vi "Marginal Condition.vi"() -> ()   [LabVIEW 2023]
doc: "This example shows how to compute the marginal condition of a spectrogram with the TFA Marginal Integration VI. The Wigner-Ville distribution (WVD) or Choi-Williams distribution (CWD) of a Gaussian chirp is computed. In theory, the time and frequency marginal conditions of the WVD and CWD are exactly corresponding to the instantaneous power and the FFT-based power spectrum respectively. The example demonstrates such property of the WVD and CWD.\n\n<b>Instructions:</b>\n1) Run this VI.\n2) Compare the <b>Power Spectrum</b> and <b>Instantaneous Power</b> of the simulated signal."
uses:
  <vilib>/Analysis/2dsp.llb/Complex FFT.vi
  <vilib>/addons/Time Frequency Analysis/Spectrogram.llb/TFA Wigner-Ville Distribution (Complex).vi
  <vilib>/addons/Time Frequency Analysis/Spectrogram.llb/TFA Choi-Williams Distribution (Complex).vi
  <vilib>/addons/Time Frequency Analysis/_control.llb/TFA Configure Spectrogram Indicator (Predefined Color Table).vi
  <vilib>/addons/_Advanced Signal Processing/NI_AdvSigProcTFA.lvlib
  <vilib>/Analysis/NI_AALPro.lvlib
panel:
  out "aspt-left-top":bool
  in  "Type":u16(ring) items=["WVD", "CWD"]
  out "Spectrogram":dbl[][](graph)
  out "Signal":cluster{"sampling rate":dbl, dbl, dbl[]}[](graph)
  out "Instantaneous power":cluster{"t0":dbl, "dt":dbl, "power":dbl[]}[](graph)
  out "Power spectrum":cluster{"f0":dbl, "df":dbl, "spectrum":dbl[]}[](graph)
  # "Overview: Shows how to compute the marginal condition of a spectrogram with the TFA Marginal Integration VI. \nRequirements: LabVIEW Full Development System, Advanced Signal Processing Toolkit\nInstructions: \n1. Run this VI.\n2. Compare the Power Spectrum and Instantaneous Power of the simulated signal."
  # "Signal and Spectrogram"
  # "Power Spectrum"
  # "Instantaneous Power"
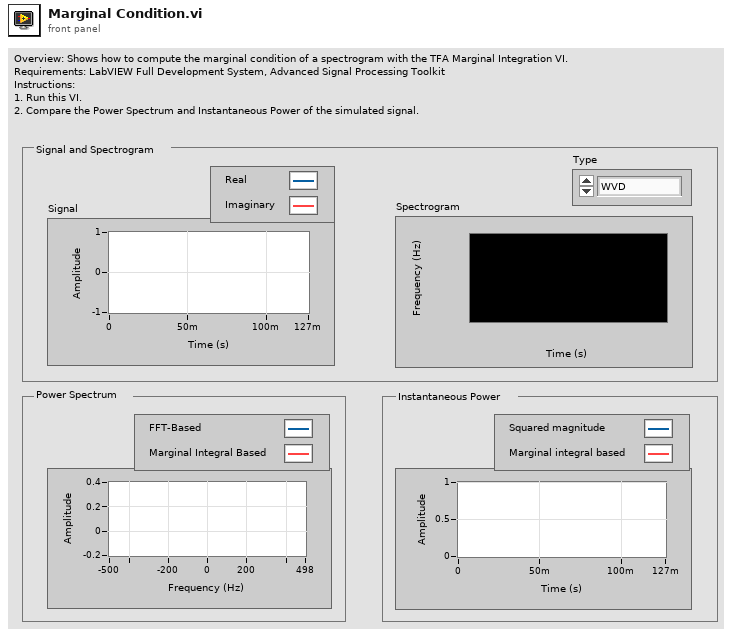
[diagram p1: front panel]
types:
  T1 = cluster{"magnitude":dbl, "phase":dbl, "std dev":dbl, "center":dbl, "frequency":dbl, "chirp rate":dbl}[]
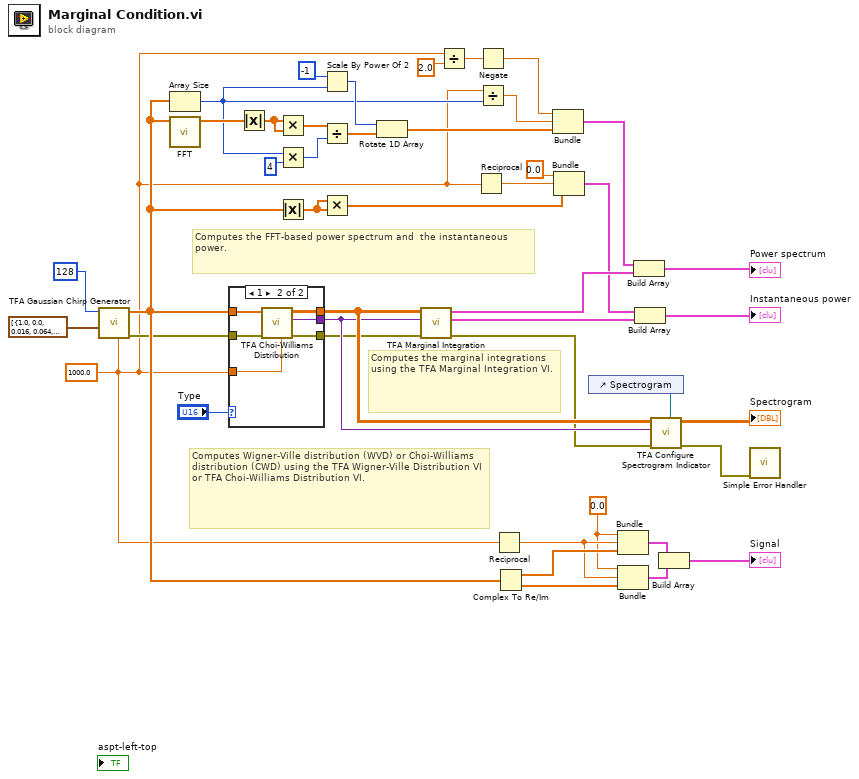
[diagram p0: block diagram]
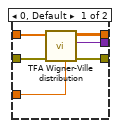
[diagram p2: hidden frame]
diagram:
  w10 = 0.0 ("sampling rate")
  w1 = 1000.0 ("sampling rate")
  # "Computes the marginal integrations using the TFA Marginal Integration VI."
  # "Computes the FFT-based power spectrum and  the instantaneous power."
  # "Computes Wigner-Ville distribution (WVD) or Choi-Williams distribution (CWD) using the TFA Wigner-Ville Distribution VI or TFA Choi-Williams Distribution VI."
  n1 = call <vilib>:"TFA Gaussian Chirp Generator.vi"("sampling rate"=w1, "chirp info"=T1 [{"magnitude"=1.0, "phase"=0.0, "std dev"=0.016, "center"=0.064, "frequency"=100.0, "chirp rate"=5000.0}] ("paras"), "samples"=128) -> ("error out"=w5:errorcluster, "Gaussian chirp"=w7:cdb[])  [unwired: 1 in, 6 out]
  n2 = Array Size(array=w7) -> (size(s)=w26:i32)
  n3 = call-poly <vilib>:"FFT.vi"("X"=w7) -> ("FFT {X}"=w43:cdb[])  [unwired: 2 in, 8 out]
  n4 = case shown="1" "Type" {
    tunnel: w7 -> [w50 w56]
    tunnel: [w49 w55] -> w32
    tunnel: [w48 w54] -> w31
    tunnel: w1 -> [w47 w53]
    tunnel: w5 -> [w46 w52]
    tunnel: [w45 w51] -> w4
    frame 0, Default {
      n5 = call-poly <vilib>:"TFA Wigner-Ville distribution.vi"("sampling rate"=w47, "error in (no error)"=w46, "signal"=w50) -> ("error out"=w45:errorcluster, "scale info"=w48:variant, "spectrogram"=w49:dbl[][])  [unwired: 1 in, 5 out]
    }
    frame 1 {
      n6 = call-poly <vilib>:"TFA Choi-Williams Distribution.vi"("sampling rate"=w53, "error in (no error)"=w52, "signal"=w56) -> ("error out"=w51:errorcluster, "scale info"=w54:variant, "spectrogram"=w55:dbl[][])  [unwired: 2 in, 4 out]
    }
  }
  n7 = Absolute Value(x=w43) -> (abs(x)=w42:dbl[])
  n8 = Multiply(x=w42, y=w42) -> (x*y=w41:dbl[])
  n9 = Multiply(x=w26, y=4) -> (x*y=w38:i32)
  n10 = Absolute Value(x=w7) -> (abs(x)=w44:dbl[])
  n11 = Scale By Power Of 2(n=-1, x=w26) -> (x*2^n=w35:i32)
  n12 = Divide(x=w41, y=w38) -> (x/y=w39:dbl[])
  n13 = Multiply(x=w44, y=w44) -> (x*y=w22:dbl[])
  n14 = Rotate 1D Array(1:w39, 2:w35) -> (0:w27:dbl[])
  n15 = call <vilib>:"TFA Marginal Integration.vi"("error in (no error)"=w4, "scale info"=w31, "spectrogram"=w32) -> ("error out"=w3:errorcluster, "time marginal integral"=w18:cluster{"t0":dbl, "dt":dbl, "power":dbl[]}, "frequency marginal integral"=w40:cluster{"f0":dbl, "df":dbl, "spectrum":dbl[]})  [unwired: 6 out]
  n16 = Divide(x=w1, y=2.0) -> (x/y=w16:dbl)
  n17 = Reciprocal(x=w1) -> (1/x=w21:dbl)
  n18 = Negate(x=w16) -> (-x=w14:dbl)
  n19 = Divide(x=w1, y=w26) -> (x/y=w25:dbl)
  n20 = Reciprocal(x=w1) -> (1/x=w11:dbl)
  n21 = Complex To Re/Im(x + iy=w7) -> (x=w13:dbl[], y=w12:dbl[])
  n22 = Bundle(w14, w25, w27) -> (w23:cluster{dbl, dbl, dbl[]})  [unwired: 1 out]
  n23 = Bundle(0.0, w21, w22) -> (w19:cluster{dbl, dbl, dbl[]})  [unwired: 1 out]
  n24 = control-ref of="Spectrogram"() -> (w29:refnum<vi>)
  n25 = Bundle("sampling rate"=w10, w11, w13) -> (w9:cluster{"sampling rate":dbl, dbl, dbl[]})  [unwired: 1 out]
  n26 = Bundle("sampling rate"=w10, w11, w12) -> (w8:cluster{"sampling rate":dbl, dbl, dbl[]})  [unwired: 1 out]
  n27 = Build Array(w23, w40) -> (→"Power spectrum":cluster{"f0":dbl, "df":dbl, "spectrum":dbl[]}[])
  n28 = Build Array(w19, w18) -> (→"Instantaneous power":cluster{"t0":dbl, "dt":dbl, "power":dbl[]}[])
  n29 = call-poly <vilib>:"TFA Configure Spectrogram Indicator.vi"("reference of TF spectrogram indicator"=w29, "error in (no error)"=w3, "scale info"=w31, "spectrogram"=w32) -> ("error out"=w2:errorcluster, "TF spectrogram indicator"=→"Spectrogram":dbl[][])  [unwired: 3 in, 3 out]
  n30 = Build Array(w9, w8) -> (→"Signal":cluster{"sampling rate":dbl, dbl, dbl[]}[])
  n31 = call <vilib>:"Simple Error Handler.vi"("error in (no error)"=w2) -> ()  [unwired: 4 in, 5 out]
